vi "OCV DMM Measure.vi"(8 "error in (no error)":errorcluster, 11 "instrument handle":refnum<k15>) -> (0 "error out":errorcluster, 1 "Voltage":sgl[](array[numeric])=[3.481668, 3.483052, 3.4783623, 3.4823976, 3.484474] format="%#_8g", 3 "refnum out":refnum<k15>, 4 "Read Time (ms)":u32=46)   [LabVIEW 2019]
uses:
  <vilib>/DAQmx/miscellaneous.llb/DAQmx Fill In Error Info.vi
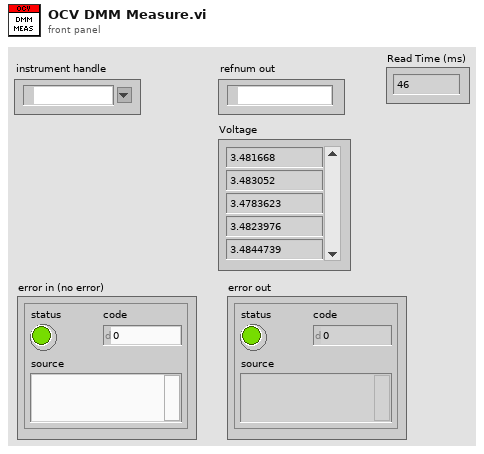
[diagram p1: front panel]
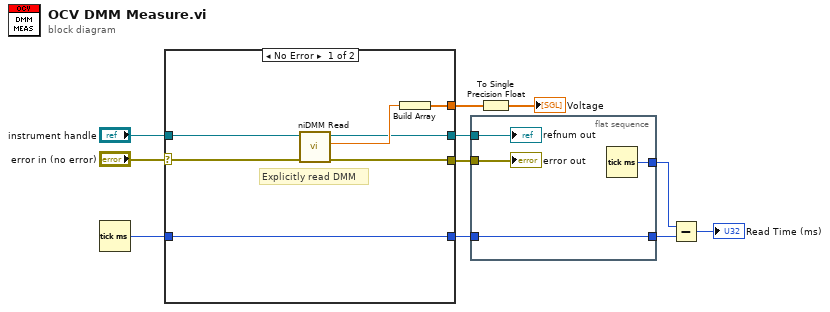
[diagram p0: block diagram]
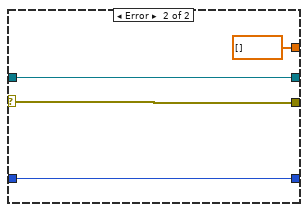
[diagram p2: hidden frame]
diagram:
  n1 = Tick Count (ms)() -> (millisecond timer value=w5:u32)
  n2 = case shown="No Error" "error in (no error)" {
    selector: "error in (no error)" -> [w16 w21]
    tunnel: [w15 sgl[] []] -> w2
    tunnel: "instrument handle" -> [w17 w22]
    tunnel: [w13 w22] -> w8
    tunnel: [w12 w21] -> w7
    tunnel: w5 -> [w18 w20]
    tunnel: [w18 w20] -> w4
    frame No Error {
      # "Explicitly read DMM"
      n3 = call <instrlib>:"niDMM Read.vi"("error in (no error)"=w16, "instrument handle"=w17) -> ("error out"=w12:errorcluster, "Measurement"=w14:dbl, "instrument handle out"=w13:refnum<k15>)  [unwired: 7 in]
      n4 = Build Array(w14) -> (w15:dbl[])
    }
    frame Error {
    }
  }
  n5 = flat-sequence {
    tunnel: [w26] -> w9
    tunnel: w4 -> [w25]
    tunnel: [w25] -> w10
    tunnel: w8 -> [w23]
    tunnel: w7 -> [w24]
    frame #0 {
      n6 = Tick Count (ms)() -> (millisecond timer value=w26:u32)
      "error out" <- w24
      "refnum out" <- w23
    }
  }
  n7 = To Single Precision Float(number=w2) -> (single precision float=→"Voltage":sgl[])
  n8 = Subtract(x=w9, y=w10) -> (x-y=→"Read Time (ms)":u32)
